vi "Interactive Test Stats.vi"() -> ()   [LabVIEW 2021]
uses:
  I64/Stats_I64_CIF_U.lvclass/Stats_I64_CIF_U.ctl
  DBL/Stats_DBL_CIF_U.lvclass/Stats_DBL_CIF_U.ctl
  858c1288-b617-4423-870e-a6a901ad366d.vi
  c5adaaea-5a1e-4328-8f42-33976745a0fd.vi
  e1c1612e-067e-4af3-8730-405ec33371b5.vi
  Time/System Time/Get System Time.vi
  DBL/New Element.vi/dfabcf33-0dbc-4041-80a5-3dc0c86d2989.vi
  DBL/X1 minus X0.vi/dfabcf33-0dbc-4041-80a5-3dc0c86d2989.vi
  DBL/Cyclic.vi/03803d02-fa6b-4a5c-be27-3f29921d93d2.vi
  I64/New Element.vi/dfabcf33-0dbc-4041-80a5-3dc0c86d2989.vi
  I64/X1 minus X0.vi/dfabcf33-0dbc-4041-80a5-3dc0c86d2989.vi
  I64/Cyclic.vi/dfabcf33-0dbc-4041-80a5-3dc0c86d2989.vi
  Time/System Time/LabVIEW Time to TAI Time.vi
  DBL/New Element.vi/dfabcf33-0dbc-4041-80a5-3dc0c86d2989.vi/9eb60a9a-770f-4d2d-8b3f-8465c267ecc9.vi
  DBL/X1 minus X0.vi/dfabcf33-0dbc-4041-80a5-3dc0c86d2989.vi/9eb60a9a-770f-4d2d-8b3f-8465c267ecc9.vi
  DBL/Cyclic.vi/03803d02-fa6b-4a5c-be27-3f29921d93d2.vi/9eb60a9a-770f-4d2d-8b3f-8465c267ecc9.vi
  I64/New Element.vi/dfabcf33-0dbc-4041-80a5-3dc0c86d2989.vi/9eb60a9a-770f-4d2d-8b3f-8465c267ecc9.vi
  I64/X1 minus X0.vi/dfabcf33-0dbc-4041-80a5-3dc0c86d2989.vi/9eb60a9a-770f-4d2d-8b3f-8465c267ecc9.vi
  I64/Cyclic.vi/dfabcf33-0dbc-4041-80a5-3dc0c86d2989.vi/9eb60a9a-770f-4d2d-8b3f-8465c267ecc9.vi
  I64/Stats_I64_CIF_U.lvclass
  DBL/Stats_DBL_CIF_U.lvclass
panel:
  out "Max Cycle dbl":dbl
  out "Average Cycle dbl":dbl
  out "Min Cycle dbl":dbl
  out "Max wait dbl":dbl
  out "Average wait dbl":dbl
  out "Min wait dbl":dbl
  out "Max Element dbl":dbl
  out "Average Element dbl":dbl
  out "Min Element dbl":dbl
  in  "Wait":u32=500
  out "Max Element":i64
  out "Average Element":dbl
  out "Min Element":i64
  out "Max wait":i64
  out "Average wait":dbl
  out "Min wait":i64
  in  "Reinit":bool
  out "Min Cycle":i64
  out "Average Cycle":dbl
  out "Max Cycle":i64
  in  "Cycle Adder":u32
  in  "stop":bool
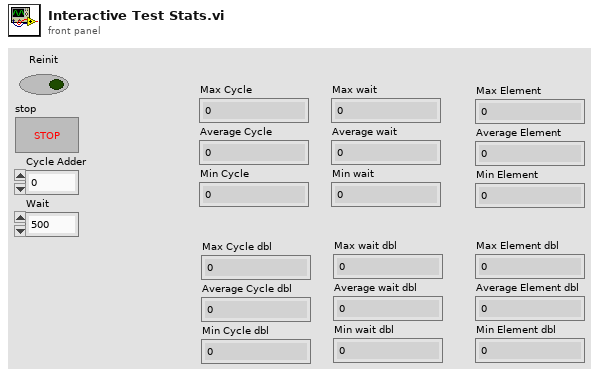
[diagram p1: front panel]
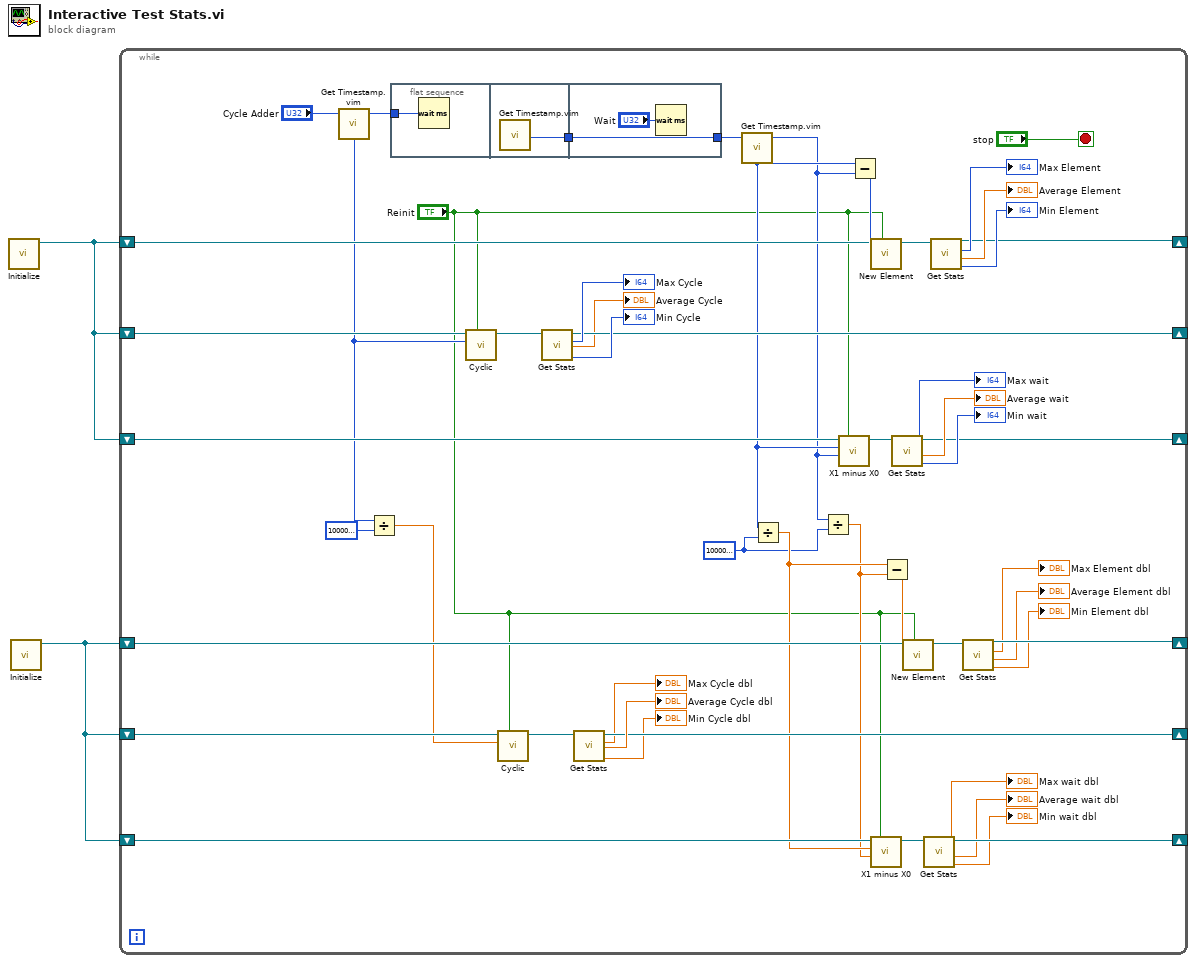
[diagram p0: block diagram]
diagram:
  n1 = call "Initialize.vi"() -> ("Stats_I64_CIF_U out"=w2:refnum<class "Stats_I64_CIF_U.lvclass">)  [unwired: 10 in, 1 out]
  n2 = call "Initialize.vi"() -> ("Stats_DBL_CIF_U out"=w1:refnum<class "Stats_DBL_CIF_U.lvclass">)  [unwired: 10 in, 1 out]
  n3 = while {
    shift-right: [w47] -> _
    shift-left: w2 -> [w51]
    shift-right: [w39] -> _
    shift-left: w2 -> [w44]
    shift-right: [w32] -> _
    shift-left: w2 -> [w37]
    shift-right: [w16] -> _
    shift-left: w1 -> [w12]
    shift-right: [w22] -> _
    shift-left: w1 -> [w17]
    shift-right: [w29] -> _
    shift-left: w1 -> [w24]
    stop <- "stop" stop-if-true
    w3 = i64 1000000000 ("y")
    n4 = call "Get Timestamp.vim"("Anything in"="Cycle Adder") -> ("Time (ns)"=w11:i64, "Anything out"=w52:u32)  [unwired: 2 in]
    n5 = Divide(x=w11, y=i64 1000000000) -> (x/y=w9:dbl)
    n6 = flat-sequence {
      tunnel: w52 -> [w55]
      tunnel: [w56] -> w46
      tunnel: [w57] -> w45
      tunnel: w46 -> [w57]
      frame #0 {
        n7 = Wait (ms)(milliseconds to wait=w55) -> ()  [unwired: 1 out]
      }
      frame #1 {
        n8 = call "Get Timestamp.vim"() -> ("Time (ns)"=w56:i64)  [unwired: 3 in, 1 out]
      }
      frame #2 {
        n9 = Wait (ms)(milliseconds to wait="Wait") -> ()  [unwired: 1 out]
      }
    }
    n10 = call "Cyclic.vi"("Reinit"="Reinit", "X"=w11, "Stats_I64_CIF_U in"=w51) -> ("Stats_I64_CIF_U out"=w50:refnum<class "Stats_I64_CIF_U.lvclass">)  [unwired: 7 in, 1 out]
    n11 = call "Cyclic.vi"("Reinit"="Reinit", "X"=w9, "Stats_DBL_CIF_U in"=w12) -> ("Stats_DBL_CIF_U out"=w13:refnum<class "Stats_DBL_CIF_U.lvclass">)  [unwired: 7 in, 1 out]
    n12 = call "Get Stats.vi"("Stats_I64_CIF_U in"=w50) -> ("Min"=→"Min Cycle":i64, "Average"=→"Average Cycle":dbl, "Max"=→"Max Cycle":i64, "Stats_I64_CIF_U out"=w47:refnum<class "Stats_I64_CIF_U.lvclass">)  [unwired: 6 in, 1 out]
    n13 = call "Get Stats.vi"("Stats_DBL_CIF_U in"=w13) -> ("Min"=→"Min Cycle dbl":dbl, "Average"=→"Average Cycle dbl":dbl, "Max"=→"Max Cycle dbl":dbl, "Stats_DBL_CIF_U out"=w16:refnum<class "Stats_DBL_CIF_U.lvclass">)  [unwired: 6 in, 1 out]
    n14 = call "Get Timestamp.vim"("Anything in"=w45) -> ("Time (ns)"=w8:i64, "Anything out"=w6:i64)  [unwired: 2 in]
    n15 = Divide(x=w8, y=w3) -> (x/y=w7:dbl)
    n16 = Divide(x=w6, y=w3) -> (x/y=w5:dbl)
    n17 = call "X1 minus X0.vi"("Reinit"="Reinit", "X0"=w6, "X1"=w8, "Stats_I64_CIF_U in"=w44) -> ("Stats_I64_CIF_U out"=w40:refnum<class "Stats_I64_CIF_U.lvclass">)  [unwired: 6 in, 1 out]
    n18 = Subtract(x=w8, y=w6) -> (x-y=w38:i64)
    n19 = call "New Element.vi"("Reinit"="Reinit", "New Element"=w38, "Stats_I64_CIF_U in"=w37) -> ("Stats_I64_CIF_U out"=w33:refnum<class "Stats_I64_CIF_U.lvclass">)  [unwired: 7 in, 1 out]
    n20 = call "X1 minus X0.vi"("Reinit"="Reinit", "X0"=w5, "X1"=w7, "Stats_DBL_CIF_U in"=w17) -> ("Stats_DBL_CIF_U out"=w21:refnum<class "Stats_DBL_CIF_U.lvclass">)  [unwired: 6 in, 1 out]
    n21 = Subtract(x=w7, y=w5) -> (x-y=w23:dbl)
    n22 = call "Get Stats.vi"("Stats_I64_CIF_U in"=w40) -> ("Min"=→"Min wait":i64, "Average"=→"Average wait":dbl, "Max"=→"Max wait":i64, "Stats_I64_CIF_U out"=w39:refnum<class "Stats_I64_CIF_U.lvclass">)  [unwired: 6 in, 1 out]
    n23 = call "New Element.vi"("Reinit"="Reinit", "New Element"=w23, "Stats_DBL_CIF_U in"=w24) -> ("Stats_DBL_CIF_U out"=w28:refnum<class "Stats_DBL_CIF_U.lvclass">)  [unwired: 7 in, 1 out]
    n24 = call "Get Stats.vi"("Stats_DBL_CIF_U in"=w21) -> ("Min"=→"Min wait dbl":dbl, "Average"=→"Average wait dbl":dbl, "Max"=→"Max wait dbl":dbl, "Stats_DBL_CIF_U out"=w22:refnum<class "Stats_DBL_CIF_U.lvclass">)  [unwired: 6 in, 1 out]
    n25 = call "Get Stats.vi"("Stats_I64_CIF_U in"=w33) -> ("Min"=→"Min Element":i64, "Average"=→"Average Element":dbl, "Max"=→"Max Element":i64, "Stats_I64_CIF_U out"=w32:refnum<class "Stats_I64_CIF_U.lvclass">)  [unwired: 6 in, 1 out]
    n26 = call "Get Stats.vi"("Stats_DBL_CIF_U in"=w28) -> ("Min"=→"Min Element dbl":dbl, "Average"=→"Average Element dbl":dbl, "Max"=→"Max Element dbl":dbl, "Stats_DBL_CIF_U out"=w29:refnum<class "Stats_DBL_CIF_U.lvclass">)  [unwired: 6 in, 1 out]
  }
